vi "TDC_getFilter.vi"(5 "Channel":i32, 11 "Error In":errorcluster) -> (6 "Filter Type":i32(ring)=1 items=["None", "Mute", "Coinc", "Sync", "Invalid"], 10 "Channel Mask":i32, 15 "Error Out":errorcluster)   [LabVIEW 2011]
uses:
  tdcbase.dll
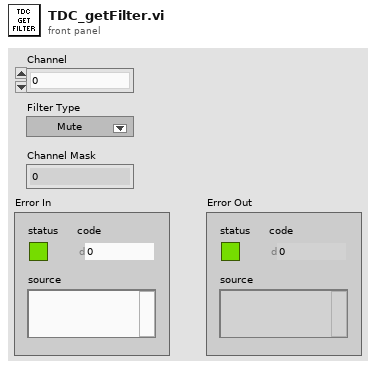
[diagram p1: front panel]
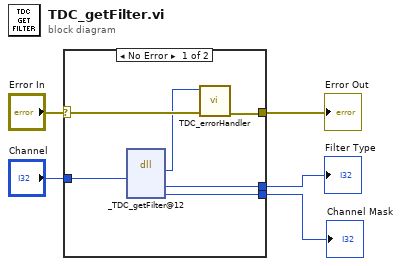
[diagram p0: block diagram]
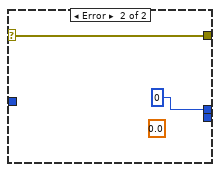
[diagram p2: hidden frame]
diagram:
  n1 = case shown="No Error" "Error In" {
    selector: "Error In" -> [w11 w13]
    tunnel: [w10 w13] -> w4
    tunnel: "Channel" -> [w8 _]
    tunnel: [w7 0] -> w2
    tunnel: [w6 _] -> w1
    frame No Error {
      n2 = dll-call lib="X:/tdcbase.dll" fn="_TDC_getFilter@12"("channel"=w8) -> ("return type"=w9:i32, "filterType"=w7:i32, "channelMask"=w6:i32)  [unwired: 6 in, 2 out]
      n3 = call "TDC_errorHandler.vi"("Error In"=w11, "TDC Return Code"=w9) -> ("Error Out"=w10:errorcluster)  [unwired: 9 in]
    }
    frame Error {
      (unwired) 0.0
    }
  }
  "Error Out" <- w4
  "Filter Type" <- w2
  "Channel Mask" <- w1
